vi "Get NamedBundler Input.vi"(8 "error in (no error)":errorcluster, 10 "Input name":string, 11 "NamedBundler ref in":refnum<vi>) -> (0 "error out":errorcluster, 1 "Found?":bool, 2 "Input Term ref":refnum<vi>, 3 "NamedBundler ref out":refnum<vi>)   [LabVIEW 2019, in "gRPC Scripting Tools.lvlib"]
uses:
  gRPC Scripting Tools.lvlib
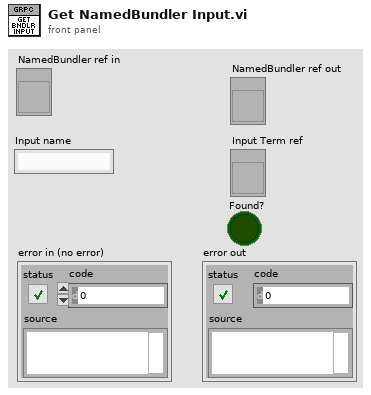
[diagram p1: front panel]
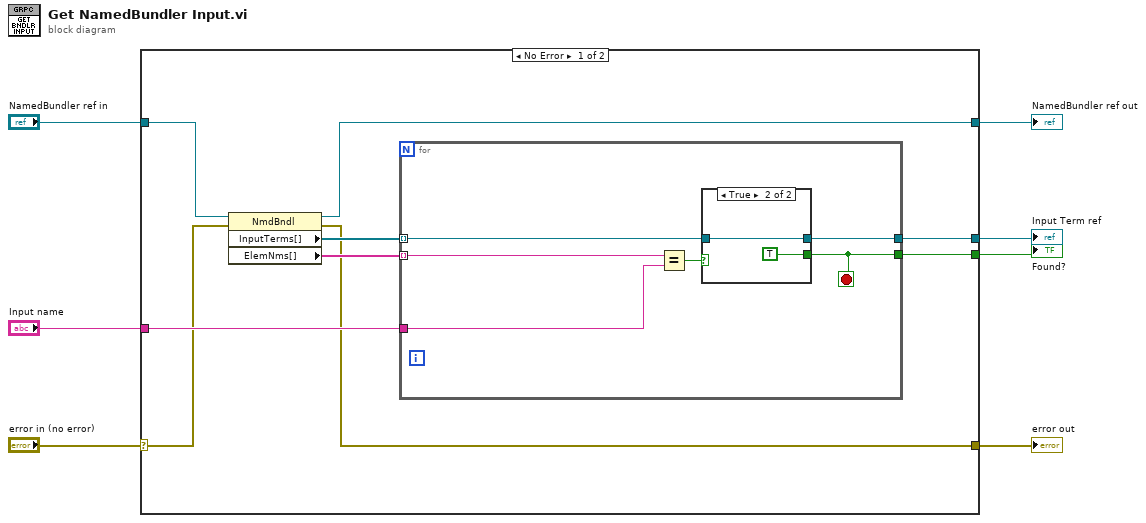
[diagram p0: block diagram]
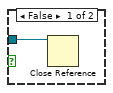
[diagram p2: hidden frame]
diagram:
  n1 = case shown="No Error" "error in (no error)" {
    selector: "error in (no error)" -> [w9 w27]
    tunnel: "Input name" -> [w16 _]
    tunnel: [w8 w27] -> w6
    tunnel: "NamedBundler ref in" -> [w12 w26]
    tunnel: [w13 _] -> w3
    tunnel: [w10 w26] -> w2
    tunnel: [w11 _] -> w1
    frame No Error {
      n2 = property class="NmdBndl"(reference=w12, error in=w9) -> (reference out=w10:refnum<vi>, error out=w8:errorcluster, "InputTerms[]"=w14:refnum<vi>[], "ElemNms[]"=w15:string[])
      n3 = for {
        tunnel: w16 -> [w22]
        tunnel: [w17] -> w11
        tunnel: w15 -> [w20] mode=indexing
        tunnel: w14 -> [w19] mode=indexing
        tunnel: [w18] -> w13
        stop <- w17 stop-if-true
        n4 = Equal?(x=w20, y=w22) -> (x = y?=w21:bool)
        n5 = case shown="True" w21 {
          tunnel: [_ TRUE] -> w17
          tunnel: w19 -> [w23 w24]
          tunnel: [_ w24] -> w18
          frame False {
            n6 = Close Reference(reference=w23) -> ()  [unwired: 1 in, 1 out]
          }
          frame True {
          }
        }
      }
    }
    frame Error {
    }
  }
  "error out" <- w6
  "NamedBundler ref out" <- w2
  "Input Term ref" <- w3
  "Found?" <- w1
